vi "Serian_Sorteddata_out.vi"(9 "Save":bool=TRUE, 10 "Cluster":T2={"Termination Character"=10, "End Read on"=TRUE, "VISA resource name"="COM1", "baud rate"=9600, "data bits"=8, "parity"=enum."None", "stop bits"=10, "flow control"=0, "XON"=enum."DC1", "XOFF"=enum."DC3", "End Write on"=TRUE} {"Termination Character" format="%.0x"; "flow control" items=["None"=0, "XON/XOFF"=1, "RTS/CTS"=2, "DTR/DSR"=4]; "data bits" min=5 max=8 step=1; "stop bits" items=["1.0"=10, "1.5"=15, "2.0"=20]; "baud rate" items=["75"=75, "110"=110, "134"=134, "150"=150, "300"=300, "600"=600, "1200"=1200, "1800"=1800, "2400"=2400, "4800"=4800, "7200"=7200, "9600"=9600, "14400"=14400, "19200"=19200, "28800"=28800, "38400"=38400, "56000"=56000, "57600"=57600, "115200"=115200, "128000"=128000, "230400"=230400]}, 11 "File_name":string="Default") -> (0 "MAIN STOP OUT":bool)   [LabVIEW 2016]
uses:
  Typedef/MCU_addresses.ctl
  Typedef/Serial_config_cluster.ctl
  Typedef/Type_of_message_to_MCU.ctl
  <vilib>/Instr/_visa.llb/VISA Configure Serial Port (Instr).vi
  <vilib>/Utility/file.llb/Write Delimited Spreadsheet (DBL).vi
panel:
  in  "MAIN STOP":bool
  in  "Types of Data":T1
  out "concatenated string":string
  out "path 2":path
  out "path":path
  out "error out 2":errorcluster
  in  "FIltering":bool
  in  "y":dbl=15.0 format="%#_13g"
  in  "index 3":i32
  in  "index 2":i32
  in  "index":i32
  out "Waveform Chart":dynamicdata(graph)
  out "Array":dbl[](array[numeric])
  in  "Read Count":u32=1000
  in  "MCU Address to be sent":T3
  in  "Payload  Byte to be sent":u8[](array[numeric])
  out "Byte array has been sent":u8[](array[numeric])
  in  "Read":bool=TRUE
  in  "Write":bool
  out "Bytes at Serial Port":u32
  out "String":string
  in  "Stop":bool
  out "Extracted Numbers":dbl[](array[numeric]) format="%#.6g"
  out "error out":errorcluster
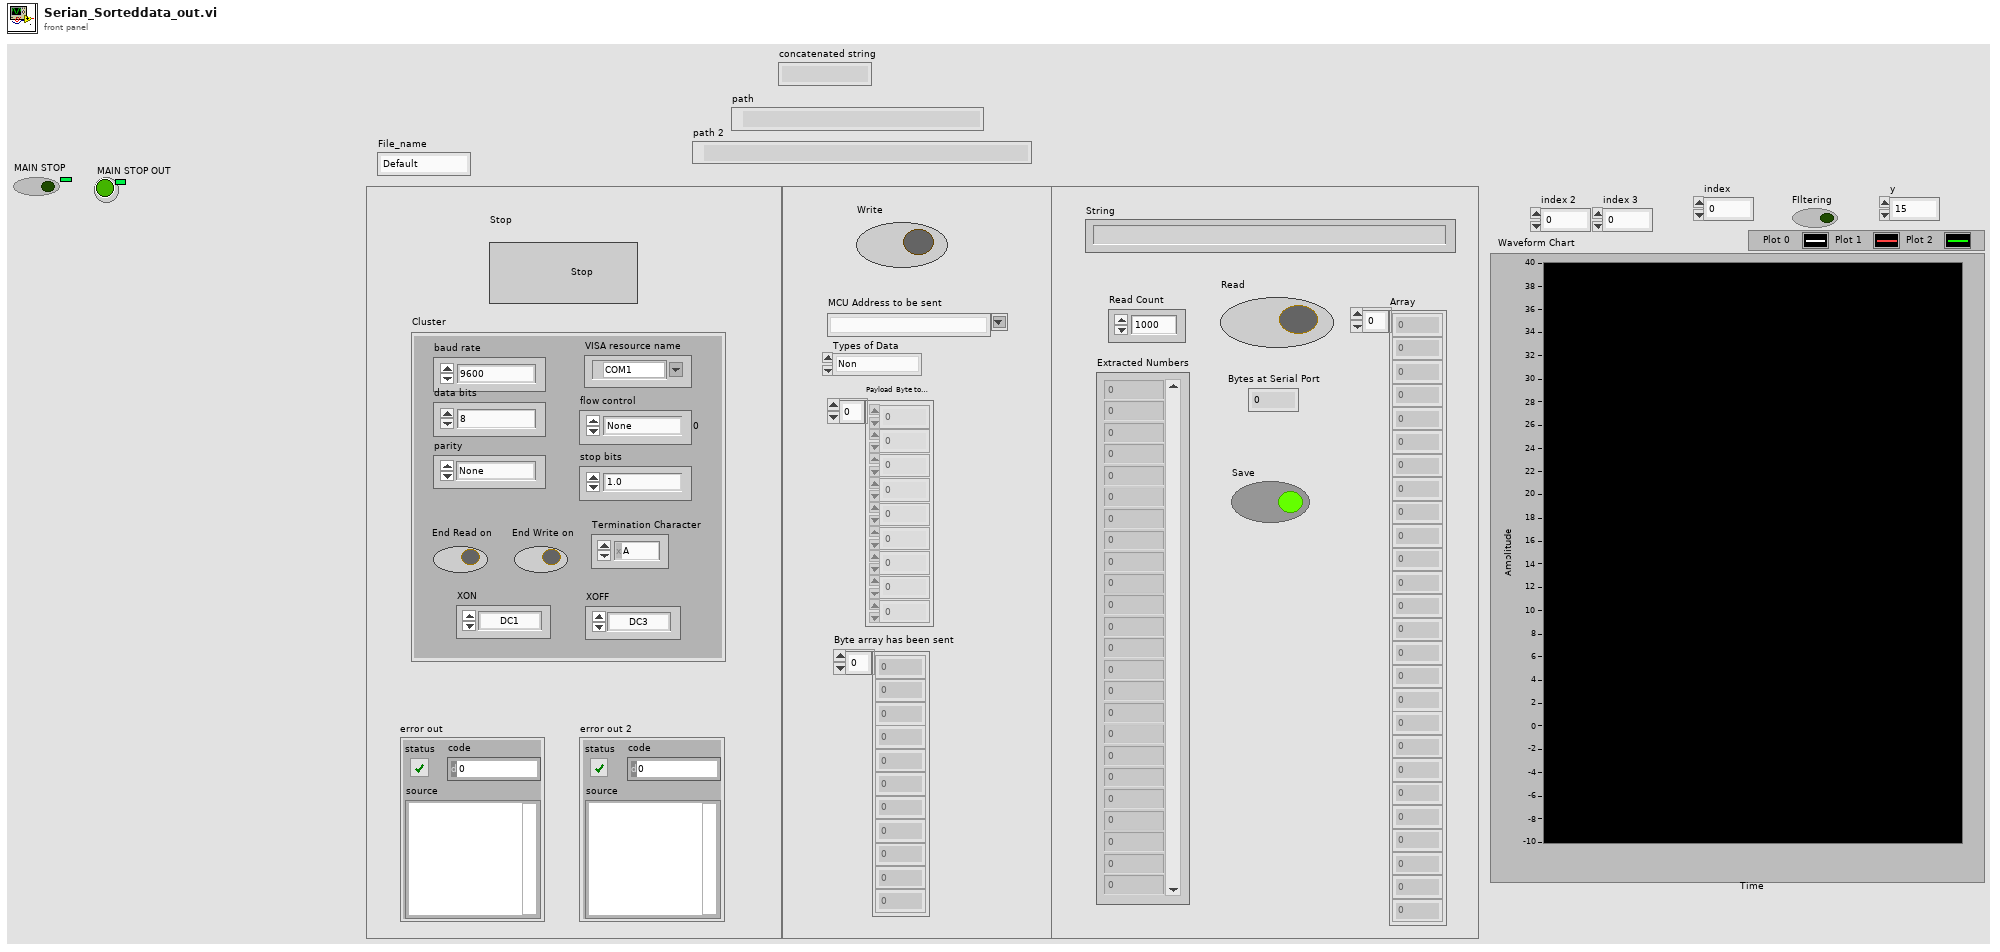
[diagram p1: front panel]
types:
  T1 = typedef "Type_of_message_to_MCU.ctl" = enum16{"Non", "Alarm", "Error", "Time and Date", "Status", "Request", "Command"}
  T2 = typedef "Serial_config_cluster.ctl" = cluster{"Termination Character":u8, "End Read on":bool, "VISA resource name":refnum<visa-resource-name>, "baud rate":u32, "data bits":u16, "parity":enum16{"None", "Odd", "Even", "Mark", "Space"}, "stop bits":u16, "flow control":u16, "XON":enum16{"NUL", "SOH", "STX", "ETX", "EOT", "ENQ", "ACK", "BEL", "BS", "HT", "LF", "VT", "FF", "CR", "SO", "SI", "DLE", "DC1", "DC2", "DC3", "DC4", "NAK", "SYN", "ETB", "CAN", "EM", "SUB", "ESC", "FS", "GS", "RS", "US", "SP", "!", "\"", "#", "$", "%", "&", "'", "(", ")", "*", "+", ",", "- (-)", ".", "/", "0", "1", "2", "3", "4", "5", "6", "7", "8", "9", ":", ";", "<", "=", ">", "?", "@", "A", "B", "C", "D", "E", "F", "G", "H", "I", "J", "K", "L", "M", "N", "O", "P", "Q", "R", "S", "T", "U", "V", "W", "X", "Y", "Z", "[", "\\", "]", "^", "_", "`", "a", "b", "c", "d", "e", "f", "g", "h", "i", "j", "k", "l", "m", "n", "o", "p", "q", "r", "s", "t", "u", "v", "w", "x", "y", "z", "{", "|", "}", "~"}, "XOFF":enum16{"NUL", "SOH", "STX", "ETX", "EOT", "ENQ", "ACK", "BEL", "BS", "HT", "LF", "VT", "FF", "CR", "SO", "SI", "DLE", "DC1", "DC2", "DC3", "DC4", "NAK", "SYN", "ETB", "CAN", "EM", "SUB", "ESC", "FS", "GS", "RS", "US", "SP", "!", "\"", "#", "$", "%", "&", "'", "(", ")", "*", "+", ",", "- (-)", ".", "/", "0", "1", "2", "3", "4", "5", "6", "7", "8", "9", ":", ";", "<", "=", ">", "?", "@", "A", "B", "C", "D", "E", "F", "G", "H", "I", "J", "K", "L", "M", "N", "O", "P", "Q", "R", "S", "T", "U", "V", "W", "X", "Y", "Z", "[", "\\", "]", "^", "_", "`", "a", "b", "c", "d", "e", "f", "g", "h", "i", "j", "k", "l", "m", "n", "o", "p", "q", "r", "s", "t", "u", "v", "w", "x", "y", "z", "{", "|", "}", "~"}, "End Write on":bool}
  T3 = typedef "MCU_addresses.ctl" = string
  T4 = enum16{"NUL", "SOH", "STX", "ETX", "EOT", "ENQ", "ACK", "BEL", "BS", "HT", "LF", "VT", "FF", "CR", "SO", "SI", "DLE", "DC1", "DC2", "DC3", "DC4", "NAK", "SYN", "ETB", "CAN", "EM", "SUB", "ESC", "FS", "GS", "RS", "US", "SP", "!", "\"", "#", "$", "%", "&", "'", "(", ")", "*", "+", ",", "- (-)", ".", "/", "0", "1", "2", "3", "4", "5", "6", "7", "8", "9", ":", ";", "<", "=", ">", "?", "@", "A", "B", "C", "D", "E", "F", "G", "H", "I", "J", "K", "L", "M", "N", "O", "P", "Q", "R", "S", "T", "U", "V", "W", "X", "Y", "Z", "[", "\\", "]", "^", "_", "`", "a", "b", "c", "d", "e", "f", "g", "h", "i", "j", "k", "l", "m", "n", "o", "p", "q", "r", "s", "t", "u", "v", "w", "x", "y", "z", "{", "|", "}", "~"}
  T5 = typedef "Message_info.ctl" = enum16{"Non", "Earthquake", "Fire", "Lost Power", "New", "Restarted"}
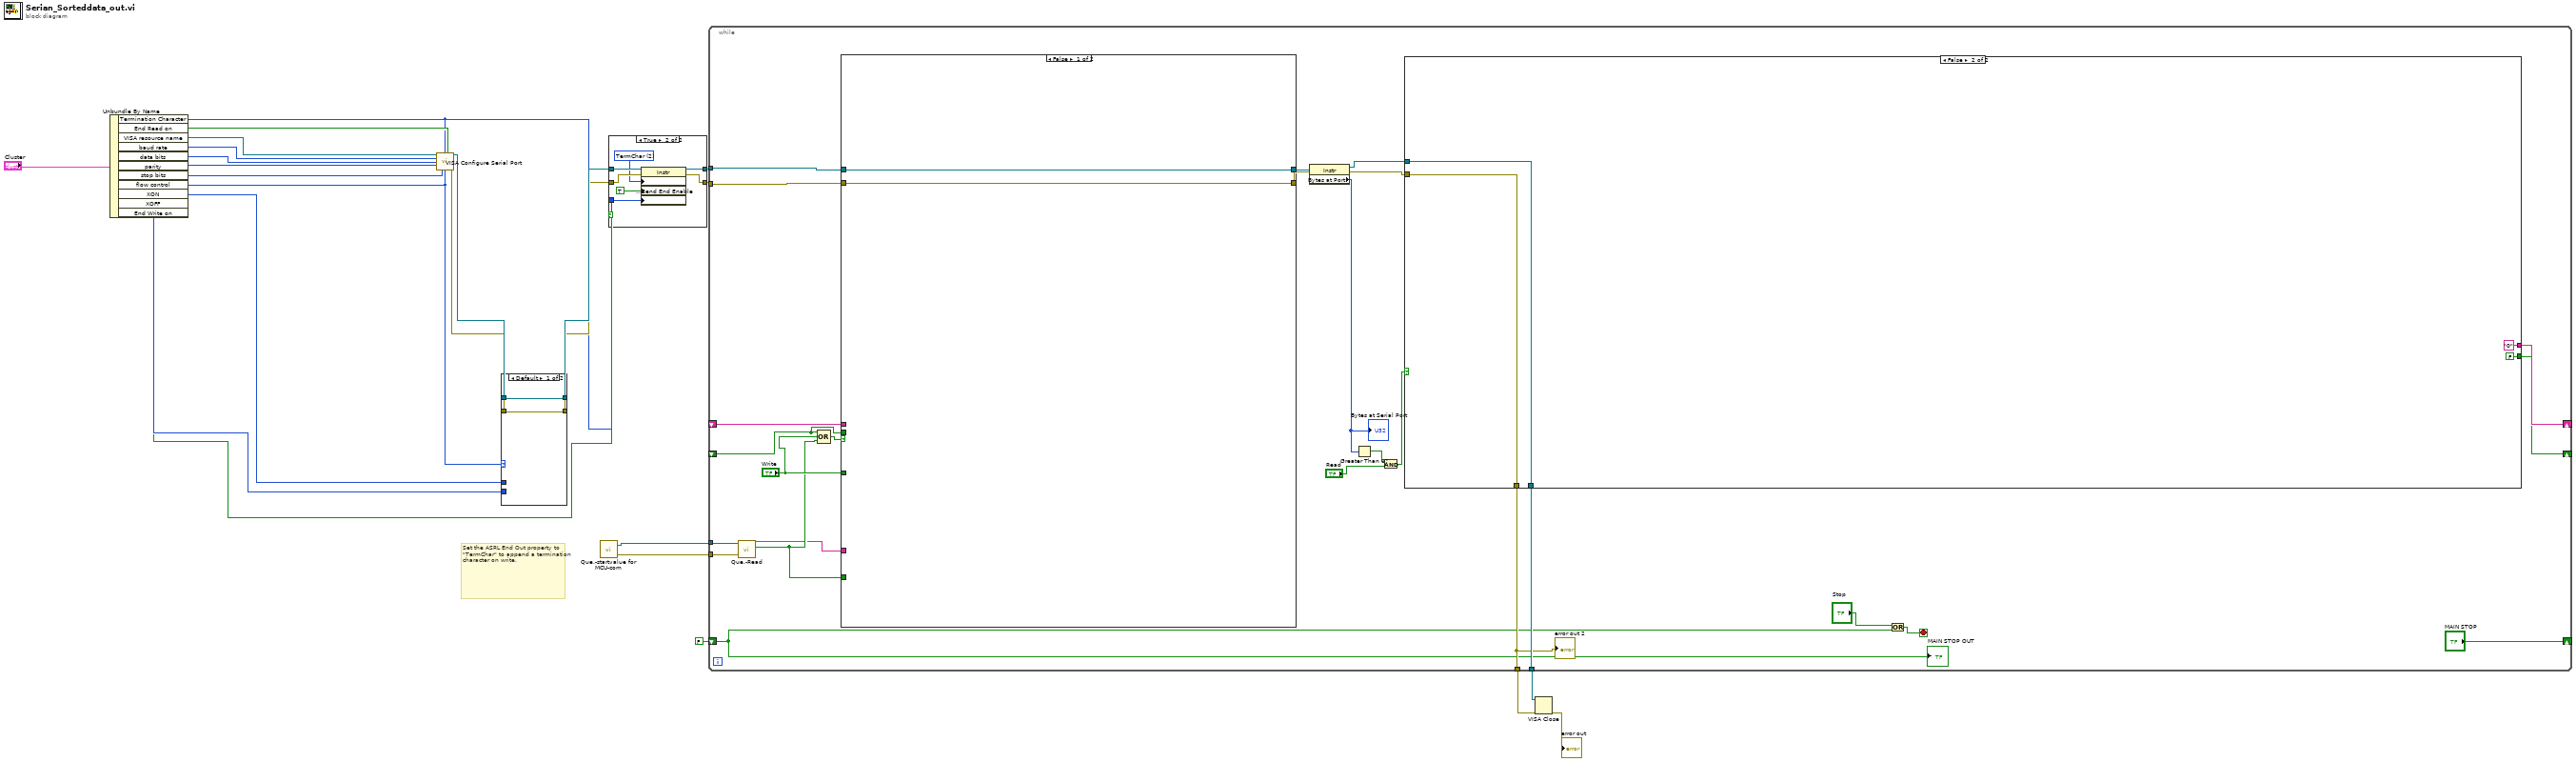
[diagram p0: block diagram]
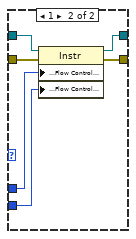
[diagram p3: hidden frame]
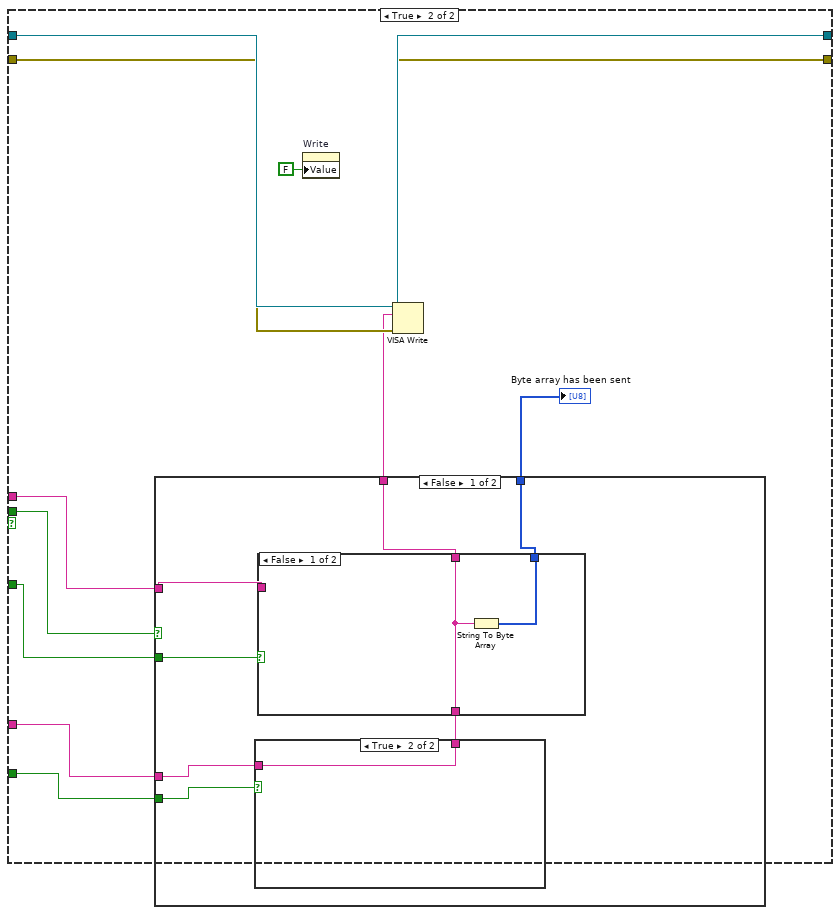
[diagram p4: hidden frame]
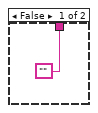
[diagram p5: hidden frame]
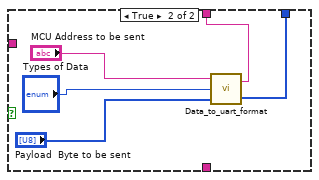
[diagram p6: hidden frame]
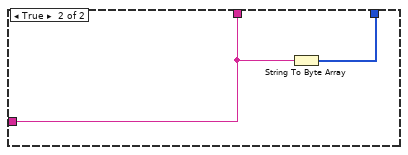
[diagram p7: hidden frame]
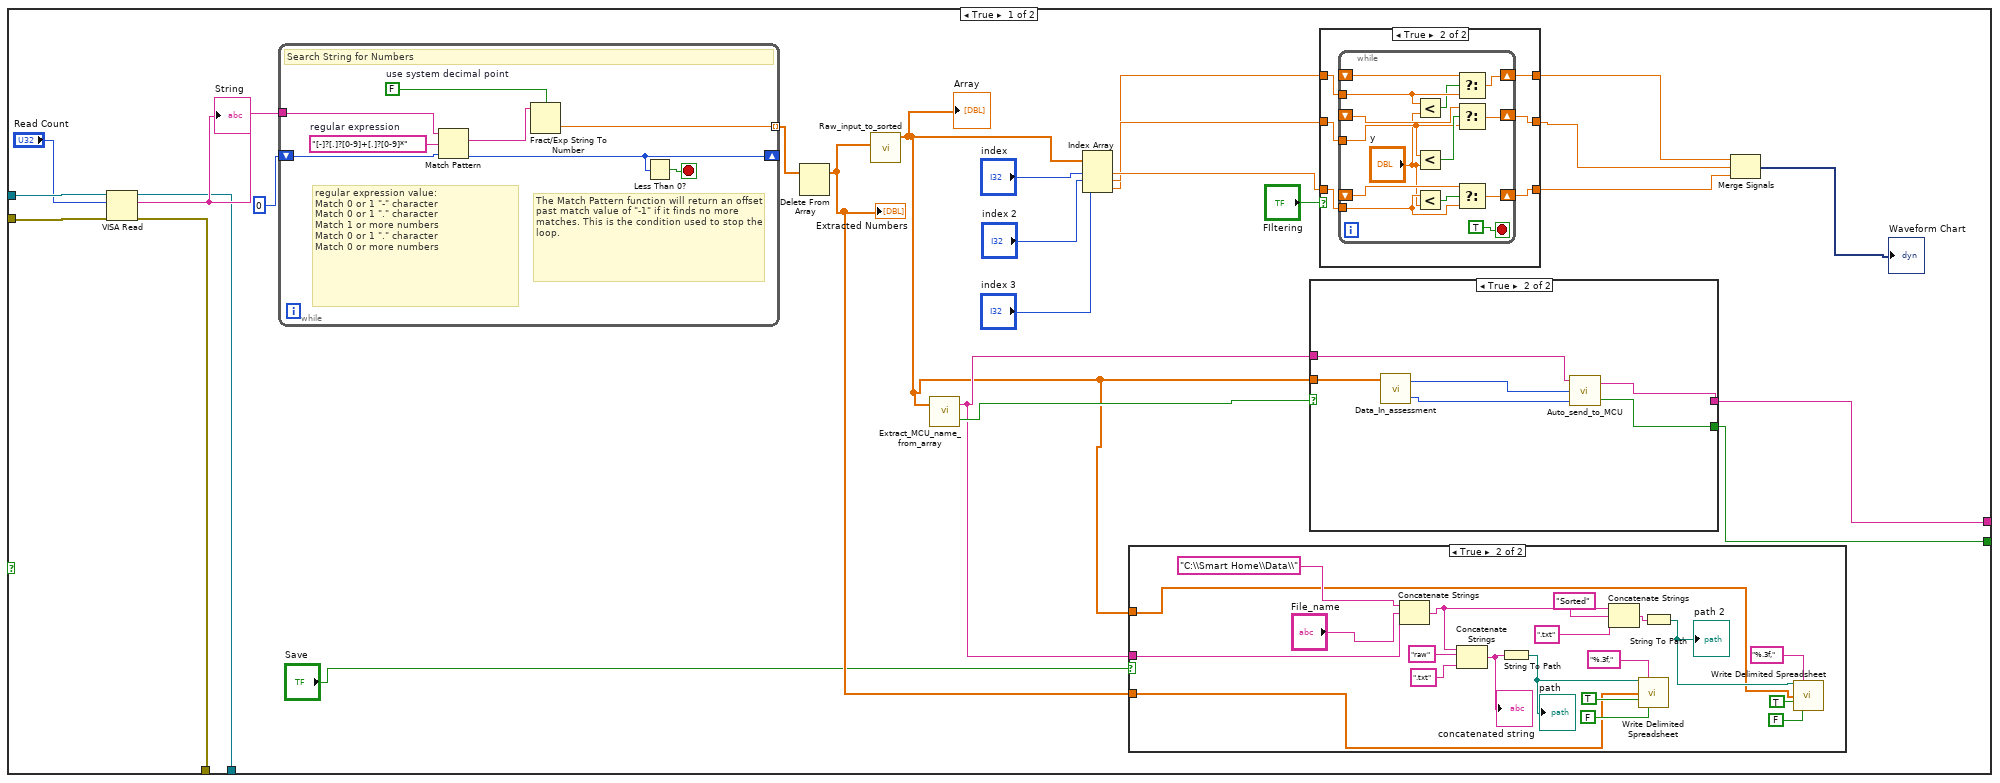
[diagram p8: hidden frame]
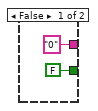
[diagram p9: hidden frame]
diagram:
  # "Set the ASRL End Out property to \"TermChar\" to append a termination character on write."
  n1 = Unbundle By Name("Cluster") -> ("Termination Character"=w4:u8, "End Read on"=w13:bool, "VISA resource name"=w14:refnum<visa-resource-name>, "baud rate"=w12:u32, "data bits"=w11:u16, "parity"=w10:enum16{"None", "Odd", "Even", "Mark", "Space"}, "stop bits"=w9:u16, "flow control"=w8:u16, "XON"=w7:T4, "XOFF"=w6:T4, "End Write on"=w5:bool)
  n2 = call-poly "VISA Configure Serial Port"("VISA resource name"=w14, "termination char\n(0xA = '\\n' = LF)"=w4, "Enable Termination\nChar (T)"=w13, "baud rate (9600)"=w12, "data bits (8)"=w11, "parity (0:none)"=w10, "stop bits (10: 1 bit)"=w9, "flow control (0:none)"=w8) -> ("VISA resource name out"=w22:refnum<visa-resource-name>, "error out"=w21:errorcluster)  [unwired: 2 in, 4 out]
  n3 = case shown="Default" w8 {
    tunnel: [w25 w32] -> w23
    tunnel: [w26 w31] -> w24
    tunnel: w21 -> [w25 w30]
    tunnel: w22 -> [w26 w29]
    tunnel: w7 -> [_ w28]
    tunnel: w6 -> [_ w27]
    frame Default {
    }
    frame 1 {
      n4 = property class="Instr"(reference=w29, error in=w30, "Serial Settings:Flow Control XON Character"=w28, "Serial Settings:Flow Control XOFF Character"=w27) -> (reference out=w31:refnum<visa-resource-name>, error out=w32:errorcluster)
    }
  }
  n5 = call "Que.-startvalue for MCU-com.vi"() -> ("error out"=w2:errorcluster, "queue out"=w3:refnum<queue>)  [unwired: 2 in]
  n6 = case shown="True" w5 {
    tunnel: w24 -> [w33 w41]
    tunnel: w23 -> [w34 w40]
    tunnel: [w33 w39] -> w20
    tunnel: [w34 w38] -> w19
    tunnel: w4 -> [_ w36]
    frame False {
    }
    frame True {
      w37 = u16 2 items=["None", "LastBit", "TermChar", "Break"] ("Serial Settings:Serial End Mode for Writes")
      n7 = property class="Instr"(reference=w41, error in=w40, "Serial Settings:End Mode for Writes"=w37, "Message Based Settings:Send End Enable"=TRUE, "Message Based Settings:Termination Character"=w36) -> (reference out=w39:refnum<visa-resource-name>, error out=w38:errorcluster)
    }
  }
  n8 = while {
    tunnel: w20 -> [w60]
    tunnel: w19 -> [w59]
    tunnel: [w57] -> w17
    tunnel: [w56] -> w16
    shift-right: [w55] -> _
    shift-left: _ -> [w53]
    shift-right: [w54] -> _
    shift-left: _ -> [w51]
    tunnel: w3 -> [w47]
    tunnel: w2 -> [w46]
    shift-right: ["MAIN STOP"] -> _
    shift-left: FALSE ("MAIN STOP") -> [w42]
    stop <- w44 stop-if-true
    n9 = call "Que.-Read.vi"("error in (no error)"=w46, "Queue in"=w47) -> ("Boolean"=w49:bool, "Output String"=w48:string)  [unwired: 8 in]
    n10 = Compound Arithmetic op=OR(w51, "Write", w49) -> (w50:bool)
    n11 = case shown="False" w50 {
      tunnel: w60 -> [w69 w81]
      tunnel: w59 -> [w68 w80]
      tunnel: [w69 w79] -> w61
      tunnel: [w68 w78] -> w63
      tunnel: w53 -> [_ w76]
      tunnel: "Write" -> [_ w71]
      tunnel: w51 -> [_ w72]
      tunnel: w49 -> [_ w74]
      tunnel: w48 -> [_ w73]
      frame False {
      }
      frame True {
        n12 = case shown="False" w72 {
          tunnel: w76 -> [w88 w98]
          tunnel: [w87 w98] -> w75
          tunnel: w74 -> [w86 _]
          tunnel: w73 -> [w85 _]
          tunnel: w71 -> [w84 _]
          tunnel: [w82 w99] -> w70
          frame False {
            n13 = case shown="True" w86 {
              tunnel: w85 -> [_ w90]
              tunnel: ["" w90] -> w83
              frame False {
              }
              frame True {
              }
            }
            n14 = case shown="False" w84 {
              tunnel: [w92 w95] -> w87
              tunnel: w88 -> [_ _]
              tunnel: w83 -> [w92 _]
              tunnel: [w91 w94] -> w82
              frame False {
                n15 = String To Byte Array(string=w92) -> (unsigned byte array=w91:u8[])
              }
              frame True {
                n16 = call "Data_to_uart_format.vi"("Payload  Byte to be sent"="Payload  Byte to be sent", "Types of Data"="Types of Data", "MCU Address to be sent"="MCU Address to be sent") -> ("Byte array has been sent"=w94:u8[], "Converted Message"=w95:string)
              }
            }
          }
          frame True {
            n17 = String To Byte Array(string=w98) -> (unsigned byte array=w99:u8[])
          }
        }
        "Byte array has been sent" <- w70
        n18 = property on="Write" class="Bool (strict)"("Value"=FALSE ("Write")) -> ()  [unwired: 2 in, 2 out]
        n19 = VISA Write(VISA resource name=w81, write buffer=w75, error in (no error)=w80) -> (VISA resource name out=w79:refnum<visa-resource-name>, error out=w78:errorcluster)  [unwired: 1 out]
      }
    }
    n20 = property class="Instr"(reference=w61, error in=w63) -> (reference out=w62:refnum<visa-resource-name>, error out=w64:errorcluster, "Bytes at Port"=w65:u32)
    "Bytes at Serial Port" <- w65
    n21 = Greater Than 0?(x=w65) -> (x > 0?=w67:bool)
    n22 = And(x=w67, y="Read") -> (x .and. y?=w58:bool)
    n23 = case shown="False" w58 {
      tunnel: w62 -> [w125 w188]
      tunnel: w64 -> [w124 w187]
      tunnel: [w118 w188] -> w57
      tunnel: [w117 w187] -> w56
      tunnel: [w104 "0" ("Converted Message")] -> w55
      tunnel: [w103 FALSE ("Send/notsend")] -> w54
      frame True {
        n24 = VISA Read(VISA resource name=w125, byte count="Read Count", error in (no error)=w124) -> (VISA resource name out=w118:refnum<visa-resource-name>, read buffer=w119:string, error out=w117:errorcluster)  [unwired: 1 out]
        "String" <- w119
        n25 = while {
          tunnel: w119 -> [w184]
          shift-left: 0 -> [w182]
          shift-right: [w179] -> _
          tunnel: [w177] -> w121 mode=indexing
          stop <- w183 stop-if-true
          w181 = FALSE  # use system decimal point
          w178 = "[-]?[.]?[0-9]+[.]?[0-9]*"  # regular expression
          # "The Match Pattern function will return an offset past match value of \"-1\" if it finds no more matches. This is the condition used to stop the loop."
          # "regular expression value:\nMatch 0 or 1 \"-\" character\nMatch 0 or 1 \".\" character\nMatch 1 or more numbers\nMatch 0 or 1 \".\" character\nMatch 0 or more numbers"
          # "Search String for Numbers"
          n26 = Match Pattern(string=w184, regular expression=w178, offset (0)=w182) -> (match substring=w180:string, offset past match=w179:i32)  [unwired: 2 out]
          n27 = Fract/Exp String To Number(use system decimal point (T)=w181, string=w180) -> (number=w177:dbl)  [unwired: 2 in, 1 out]
          n28 = Less Than 0?(x=w179) -> (x < 0?=w183:bool)
        }
        n29 = Delete From Array(array=w121) -> (array with subset deleted=w122:dbl[])  [unwired: 2 in, 1 out]
        "Extracted Numbers" <- w122
        n30 = call "Raw_input_to_sorted.vi"("Input Array"=w122) -> ("Array Out"=w100:dbl[])  [unwired: 10 in]
        "Array" <- w100
        n31 = call "Extract_MCU_name_from_array.vi"("Input Array"=w100) -> ("In Range?"=w102:bool, "MCU Name"=w101:string)  [unwired: 1 in]
        n32 = Index Array(array=w100, index #1="index", index #2="index 2", index #3="index 3") -> (element #1=w112:dbl, element #2=w111:dbl, element #3=w110:dbl)
        n33 = case shown="True" "Save" {
          tunnel: w122 -> [_ w173]
          tunnel: w100 -> [_ w158]
          tunnel: w101 -> [_ w157]
          frame False {
          }
          frame True {
            n34 = Concatenate Strings("C:\\Smart Home\\Data\\", "File_name", w157) -> (w162:string)
            n35 = Concatenate Strings(w162, "raw" ("string"), ".txt") -> (w161:string)
            "concatenated string" <- w161
            n36 = String To Path(string=w161) -> (path=w168:path)
            "path" <- w168
            n37 = Concatenate Strings(w162, "Sorted" ("string"), ".txt") -> (w167:string)
            n38 = call-poly <vilib>:"Write Delimited Spreadsheet.vi"("file path (dialog if empty)"=w168, "format (%.3f)"="%.3f,", "1D data"=w173, "append to file? (new file:F)"=TRUE, "transpose? (no:F)"=FALSE) -> ()  [unwired: 9 in, 2 out]
            n39 = String To Path(string=w167) -> (path=w166:path)
            "path 2" <- w166
            n40 = call-poly <vilib>:"Write Delimited Spreadsheet.vi"("file path (dialog if empty)"=w166, "format (%.3f)"="%.3f,", "1D data"=w158, "append to file? (new file:F)"=TRUE, "transpose? (no:F)"=FALSE) -> ()  [unwired: 9 in, 2 out]
          }
        }
        n41 = case shown="True" w102 {
          tunnel: w100 -> [_ w133]
          tunnel: ["0" ("Converted Message") w130] -> w104
          tunnel: [FALSE ("Send/notsend") w129] -> w103
          tunnel: w101 -> [_ w128]
          frame False {
          }
          frame True {
            n42 = call "Data_In_assessment.vi"("Array"=w133) -> ("Message Form"=w131:T5, "Types of Data"=w132:T1)  [unwired: 1 in]
            n43 = call "Auto_send_to_MCU.vi"("Message Form"=w131, "Types of Data"=w132, "MCU Name"=w128) -> ("Send/notsend"=w129:bool, "Converted Message"=w130:string)
          }
        }
        n44 = case shown="True" "FIltering" {
          tunnel: w112 -> [w136 w142]
          tunnel: w111 -> [w135 w141]
          tunnel: w110 -> [w134 w140]
          tunnel: [w134 w138] -> w108
          tunnel: [w135 w137] -> w107
          tunnel: [w136 w139] -> w106
          frame False {
          }
          frame True {
            n45 = while {
              tunnel: w142 -> [w154]
              tunnel: w141 -> [w151]
              tunnel: w140 -> [w148]
              shift-right: [w145] -> w138
              shift-left: _ -> [w146]
              shift-right: [w150] -> w137
              shift-left: _ -> [w149]
              shift-right: [w156] -> w139
              shift-left: _ -> [w155]
              stop <- TRUE stop-if-true
              n46 = Less?(x=w148, y="y") -> (x < y?=w147:bool)
              n47 = Less?(x=w151, y="y") -> (x < y?=w152:bool)
              n48 = Less?(x=w154, y="y") -> (x < y?=w153:bool)
              n49 = Select(t=w146, s=w147, f=w148) -> (s? t:f=w145:dbl)
              n50 = Select(t=w149, s=w152, f=w151) -> (s? t:f=w150:dbl)
              n51 = Select(t=w155, s=w153, f=w154) -> (s? t:f=w156:dbl)
            }
          }
        }
        n52 = Merge Signals(w108, w107, w106) -> (→"Waveform Chart":dynamicdata)
      }
      frame False {
      }
    }
    "error out 2" <- w56
    n53 = Or(x="Stop", y=w42) -> (x .or. y?=w44:bool)
    "MAIN STOP OUT" <- w42
  }
  n54 = VISA Close(VISA resource name=w17, error in (no error)=w16) -> (error out=→"error out":errorcluster)
